vi "事件结构（按钮按下计数）.vi"() -> ()   [LabVIEW 2017]
panel:
  in  "停止":bool
  out "Count":i32
  in  "Hit Me！":bool
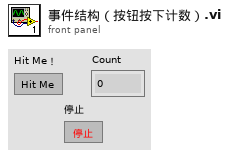
[diagram p1: front panel]
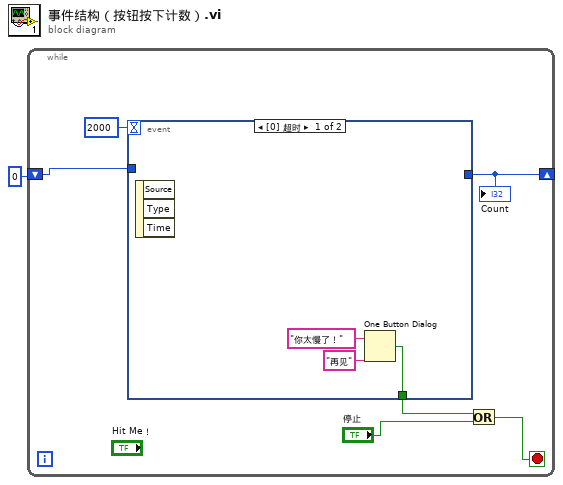
[diagram p0: block diagram]
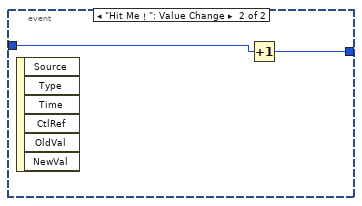
[diagram p2: hidden frame]
diagram:
  n1 = while {
    shift-right: [w5] -> _
    shift-left: 0 -> [w6]
    stop <- w4 stop-if-true
    n2 = event shown="[0] 超时" {
      selector: _ -> [_ _]
      dyn-events: _ -> [_ _]
      timeout: 2000 -> [_ _]
      tunnel: w6 -> [_ w12]
      tunnel: [_ w11] -> w5
      tunnel: [w10 _] -> w2
      event Timeout {
        n3 = event-data() -> ()  [unwired: 1 in, 3 out]
        n4 = One Button Dialog(message="你太慢了！" ("消息"), button name ("OK")="再见" ("按钮名称（“确定”）")) -> (true=w10:bool)
      }
      event "Hit Me！": Value Change {
        n5 = event-data() -> ()  [unwired: 1 in, 6 out]
        n6 = Increment(x=w12) -> (x+1=w11:i32)
      }
    }
    "Count" <- w5
    n7 = Or(x=w2, y="停止") -> (x .or. y?=w4:bool)
  }
